vi "chart series set marker fill.vi"(8 "error in (no error)":errorcluster, 10 "fill":T1, 11 "series":u32) -> (0 "error out":errorcluster, 2 "fill out":T1)   [LabVIEW 2015, in "xlsxwriter.lvlib"]
doc: "void chart_series_set_marker_fill(lxw_chart_series series, lxw_chart_fill *fill);"
uses:
  xlsxwriter.lvlib
  xlsxwriter.dll
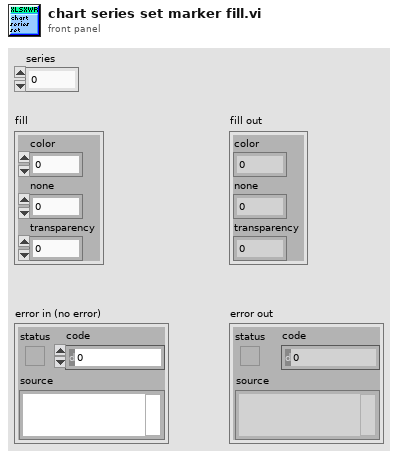
[diagram p1: front panel]
types:
  T1 = cluster{"color":u32, "none":u8, "transparency":u8}
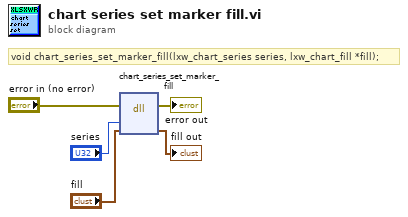
[diagram p0: block diagram]
diagram:
  # "void chart_series_set_marker_fill(lxw_chart_series series, lxw_chart_fill *fill);"
  n1 = dll-call lib="C:/Users/WDAGUtilityAccount/Desktop/lv_vis_added_cell/xlsxwriter.*" fn="chart_series_set_marker_fill"(error in="error in (no error)", "series"="series", "fill"="fill") -> (error out=→"error out":errorcluster, "fill"=→"fill out":T1)  [unwired: 4 in, 1 out]
